vi "ReadFileContent.vi"(7 "Minimum File Size":i64, 8 "error in":errorcluster, 11 "File Path":path) -> (0 "error out":errorcluster, 1 "Content":string, 3 "File Path out":path)   [LabVIEW 2021]
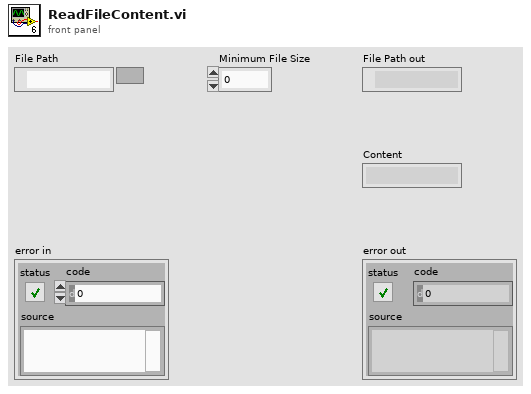
[diagram p1: front panel]
types:
  T1 = enum16{"open", "replace", "create", "open or create", "replace or create", "replace or create with confirmation"}
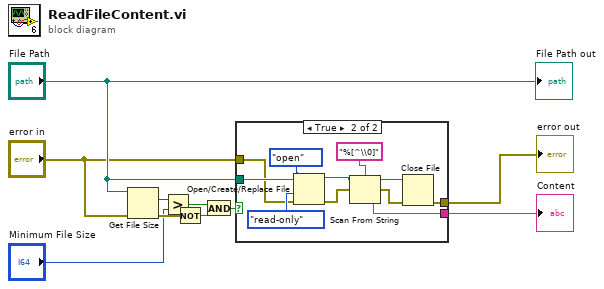
[diagram p0: block diagram]
diagram:
  n1 = Get File Size(file="File Path", error in="error in") -> (size (in bytes)=w3:i64, 0:w6:errorcluster)  [unwired: 1 out]
  n2 = Greater?(x=w3, y="Minimum File Size") -> (0:w8:bool)
  n3 = Not(x=w6) -> (.not. x?=w9:bool)
  n4 = And(x=w8, y=w9) -> (x .and. y?=w5:bool)
  n5 = case shown="True" w5 {
    tunnel: "File Path" -> [_ w16]
    tunnel: [_ w14] -> w10
    tunnel: "error in" -> [w11 w13]
    tunnel: [w11 w12] -> w1
    frame False {
    }
    frame True {
      n6 = Open/Create/Replace File(file path (use dialog)=w16, error in=w13, operation (0:open)=T1."open", access (0:read/write)=enum16{"read/write", "read-only", "write-only"}."read-only") -> (refnum out=w19:refnum<file>, error out=w20:errorcluster)  [unwired: 2 in, 1 out]
      n7 = Scan From String("%[^\\0]" ("format string"), w19, w20) -> (w22:refnum<file>, w21:errorcluster, output 1=w14:string)  [unwired: 1 in]
      n8 = Close File(refnum=w22, error in=w21) -> (error out=w12:errorcluster)  [unwired: 1 out]
    }
  }
  "Content" <- w10
  "error out" <- w1
  "File Path out" <- "File Path"
